vi "PIFN_System_GUI.vi"() -> ()   [LabVIEW 2019]
doc: "This example shows how to configure multiple channels and acquire waveforms from multiple channels."
uses:
  <vilib>/Utility/error.llb/DialogType.ctl
  <vilib>/Instr/_visa.llb/VISA Configure Serial Port (Instr).vi
  subVIs/SiPM_Tests_Global_Var.vi
  subVIs/Agilent_lib/Public/Configure/Trigger/Configure Trigger (Edge).vi
  subVIs/Agilent_lib/Agilent 2000 3000 X-Series.lvlib
panel:
  in  "Use Default Dir.":bool=TRUE
  out "Properties":string[](array[string])
  in  "Close Session":bool
  in  "HP8116A":refnum<visa-resource-name>="GPIB0::16::INSTR" caption="Function Generator HP8116A"
  in  "Power supply Agilent E3631A":refnum<visa-resource-name>="GPIB0::5::INSTR"
  out "Meas Ind":bool
  in  "x = y?":bool
  in  "Spectrum Only":bool
  in  "System Type":bool=TRUE
  in  "Nb_of_Events":i32 caption="Events to Record"
  in  "Abort":bool
  in  "Step Size (mm)":sgl=4.2 min=0 step=0.2
  in  "Nb of steps":u8=144
  in  "Nb of Events per step":u16=100
  in  "Time to Run (s)":dbl
  in  "System Settings":bool
  in  "Load file to display":bool
  in  "Calibration Tests":bool
  in  "Stop Button":bool
  in  "Free Run":bool
  in  "Tab Control 2":T1(tab)=enum."DPC System"
  in  "Trigger Source":T2(ring)
  in  "Input \nCoupling":T3(ring)=enum."DC Coupling"
  in  "Edge \nSlope":enum16{"Pos", "Neg", "Either", "Alt"}(ring)=enum."Neg"
  in  "Trigger Level (V)":dbl(knob)=-0.045 min=-10.0 max=10.0 step=0.01 scale=0.0..5.0
  in  "EN 4":bool
  in  "Ch 4 Vertical Scale":dbl(knob)=0.1 min=0.0 max=5.0 step=0.05 scale=0.0..5.0
  in  "CH 4  offset":dbl(knob)=-0.35 min=-10.0 max=10.0 step=0.01 scale=0.0..10.0
  in  "Ch3 Vertical Scale":dbl(knob)=0.1 min=0.0 max=5.0 step=0.05 scale=0.0..5.0
  in  "CH 3  offset":dbl(knob)=-0.35 min=-10.0 max=10.0 step=0.01 scale=0.0..10.0
  in  "EN 3":bool
  in  "EN 2":bool=TRUE
  in  "Ch 2 Vertical Scale":dbl(knob)=0.1 min=0.0 max=5.0 step=0.05 scale=0.0..5.0
  in  "CH 2  offset":dbl(knob)=-0.35 min=-10.0 max=10.0 step=0.01 scale=0.0..10.0
  in  "Ch1 Vertical Scale":dbl(knob)=0.1 min=0.0 max=5.0 step=0.001 scale=0.0..5.0
  in  "CH 1  offset":dbl(knob)=-0.35 min=-10.0 max=10.0 step=0.01 scale=0.0..10.0
  in  "EN":bool=TRUE
  in  "Agilent MSO-X 3104A \nOscilloscope":refnum<visa-resource-name>="USB0::0x0957::0x17A0::MY54100381::INSTR"
  out "Scope 2":waveform(dbl)[](graph)
  in  "Impedance":enum16{"1 MOhm", "50 Ohm"}(ring)=enum."50 Ohm"
  in  "Coupling":enum16{"AC", "DC"}(ring)=enum."DC"
  in  "Vertical Setting":enum16{"Vertical Scale", "Vertical Range"}(ring)
  in  "Vertical Range":dbl=40.0
  in  "Time per Division":dbl(knob)=1e-07 scale=0.0..1.0
  in  "Horizontal \nPosition":dbl(knob) scale=0.0..1.0
  in  "Ch1":u8=1 min=1 max=10 step=9
  in  "Ch2":u8=1 min=1 max=10 step=9
  in  "Ch3":u8=1 min=1 max=10 step=9
  in  "Ch4":u8=1 min=1 max=10 step=9
  in  "Trigger Source":T4(ring)
  out "Sync Error":bool
  in  "Nb of Laser Pulses":u8=1
  in  "Trig Delay":u8=50
  in  "Trig Width":u8=5
  in  "Delay":i16=30
  in  "Edge Det\nDisable":bool
  out "Spectrum":u16[][](graph)
  in  "Read Info":bool
  in  "Integr_dur":sgl(slide)=6.0 caption="Integration Duration (us)" min=0 max=12.75 step=0.05 scale=0.0..12.0 scale format="%#.2f"
  in  "Trigger thr (V)":sgl(slide)=0.005 min=0 max=3.3 step=0.001 scale=0.0..3.3
  out "Firmware Version":string="1"
  out "Hardware":string="1"
  out "Project":string="1"
  in  "DAQ Serial Port":refnum<visa-resource-name>="COM7"
  out "UART":bool
  in  "Download Confg":bool
  in  "SetSize":bool
  in  "FIFO pkt size":u16
  in  "RdFIFO 2":bool
  out "Buf Data":u8[](array[numeric])
  in  "FlushBuf":bool
  in  "RdFIFO":bool
  in  "Cmd ID":u8
  in  "Send CMD":bool
  in  "RdADC":bool
  out "ADC_data":u16
  in  "RdReg":bool
  in  "WrReg":bool
  out "RdReg_data":u8
  in  "WrReg_data":u8
  in  "RdReg_addr":u8
  in  "WrReg_addr":u8
  in  "RdReg 2":bool
  out "Bytes at port":u16
  out "Ch1":u16[](array[numeric])
  out "Ch4":u16[](array[numeric])
  out "Ch2":u16[](array[numeric])
  out "Ch3":u16[](array[numeric])
  in  "Tab Control":enum32{"Spectrum", "SiPM Array"}(tab)=enum."SiPM Array"
  in  "Spectrum?":bool
  in  "Bin Min (V)":dbl
  in  "Bin Max (V)":dbl=3.3
  out "XY Graph":T5(graph) caption="Spectrum"
  in  "Serial Settings":T6={"VISA resource name"="COM3", "baud rate"=9600, "data bits"=8, "parity"=enum."None", "stop bits"=10, "flow control"=0} {"flow control" items=["None"=0, "XON/XOFF"=1, "RTS/CTS"=2, "DTR/DSR"=4]; "stop bits" items=["1.0"=10, "1.5"=15, "2.0"=20]; "data bits" min=5 max=8 step=1}
  out "Y Position":dbl
  out "X position":dbl
  in  "Set Home":bool
  in  "Reset Stepper":bool
  out "Serial":string caption="Serial Monitor"
  in  "Motor Home":bool
  in  "Step (mm)":sgl min=0 step=0.2
  in  "X Back":bool
  in  "X forward":bool
  in  "Y back":bool
  in  "Y forward":bool
  out "en_channels":bool[](array[boolean])
  out "Col":dbl caption="Column Mean Fraction" format="%.2f"
  out "Row":dbl caption="Row Mean Fraction" format="%.2f"
  out "SiPM Y":i32 caption="SiPM Column"
  out "SiPM X":i32 caption="SiPM Row"
  out "Y-Home":dbl caption="Y-Home Position"
  out "X-Home":dbl caption="X-Home Position"
  out "Pulser":bool
  out "Bias":bool
  out "Power":bool
  out "Scope":bool
  out "Session Log":string
  in  "Read Temperature":bool
  out "Celcius":dbl(slide) scale=0.0..30.0
  in  "Default?":bool=TRUE
  out "Time (s)":dbl format="%.2f"
  in  "Save Results?":bool=TRUE
  in  "Set Manual Temp?":bool=TRUE
  in  "Temperature":string
  in  "Settings Button":bool
  in  "Results Directory":path=path "C:/Users/johnk/Desktop/ESA_Scintillator_Data"
  out "Events Recorded":i32
  in  "Measurement":string
  in  "File Name":string="1"
  in  "Enable\nVernier":bool
  in  "Enable \nREF \nBNC":bool
  in  "Time Base Type":i32(ring) items=["Main", "Window", "XY", "Roll"]
  # "NCSR  DEMOKRITOS\nInstitute of Nuclear and Particle Physics\nDetectors Instrumentation Laboratory"
  # "Proton-Ion-Fast Neutron Subsystem"
  # "Free Run Tests"
  # "Stepper Motor"
  # "Probe Attenuation"
  # "DAQ Configuration"
  # "Laser Position"
  # "Current Pos in SiPM Array"
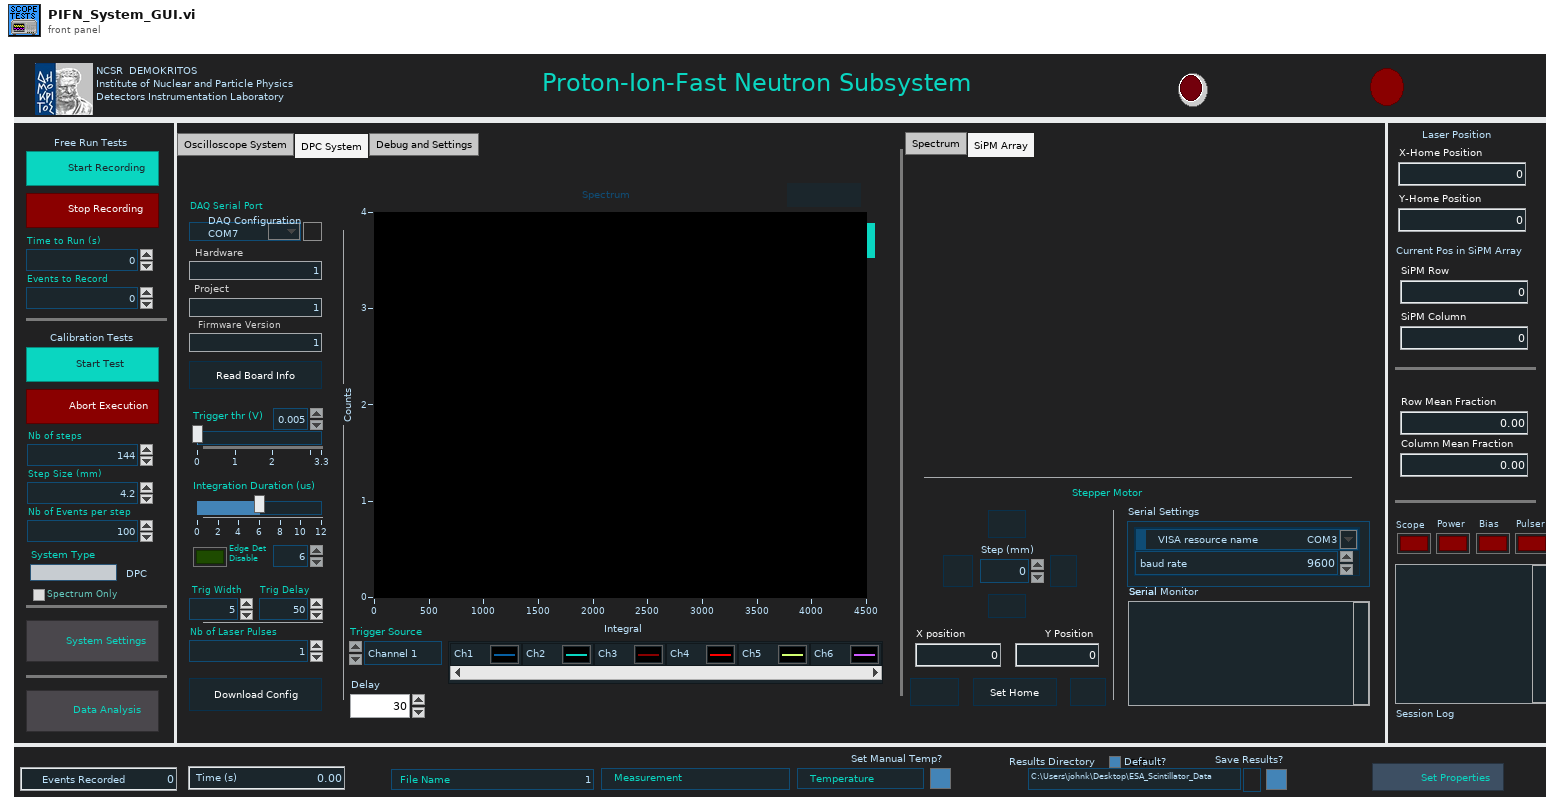
[diagram p1: front panel]
types:
  T1 = enum32{"Oscilloscope System", "DPC System", "Debug and Settings"}
  T2 = enum16{"Channel 1", "Channel 2", "Channel 3", "Channel 4", "D0", "D1", "D2", "D3", "D4", "D5", "D6", "D7", "D8", "D9", "D10", "D11", "D12", "D13", "D14", "D15", "External", "Power Line", "Waveform Generator"}
  T3 = enum16{"AC Coupling", "DC Coupling", "Low Frequency Reject"}
  T4 = enum16{"Channel 1", "Channel 2", "Channel 3", "Channel 4", "Channel 5", "Channel 6"}
  T5 = cluster{"X Values":dbl[], "Histogram: h(x)":i32[]}[]
  T6 = cluster{"VISA resource name":refnum<visa-resource-name>, "baud rate":u32, "data bits":u16, "parity":enum16{"None", "Odd", "Even", "Mark", "Space"}, "stop bits":u16, "flow control":u16}
  T7 = typedef "DialogType.ctl" = u16
  T8 = cluster{"error":bool, "code":i32, "source":string}
  T9 = enum16{"big-endian, network order", "native, host order", "little-endian"}
  T10 = enum16{"open", "open or create", "create or replace", "create", "open (read-only)"}
  T11 = cluster{"Ch1_in":dbl[], "Ch2_in":dbl[], "Ch3_in":dbl[], "Ch4_in":dbl[]}
  T12 = cluster{"Ch1":dbl[], "Ch2":dbl[], "Ch3":dbl[], "Ch4":dbl[]}
  T13 = cluster{dbl[], "mean value":dbl, dbl[], "mean value":dbl}
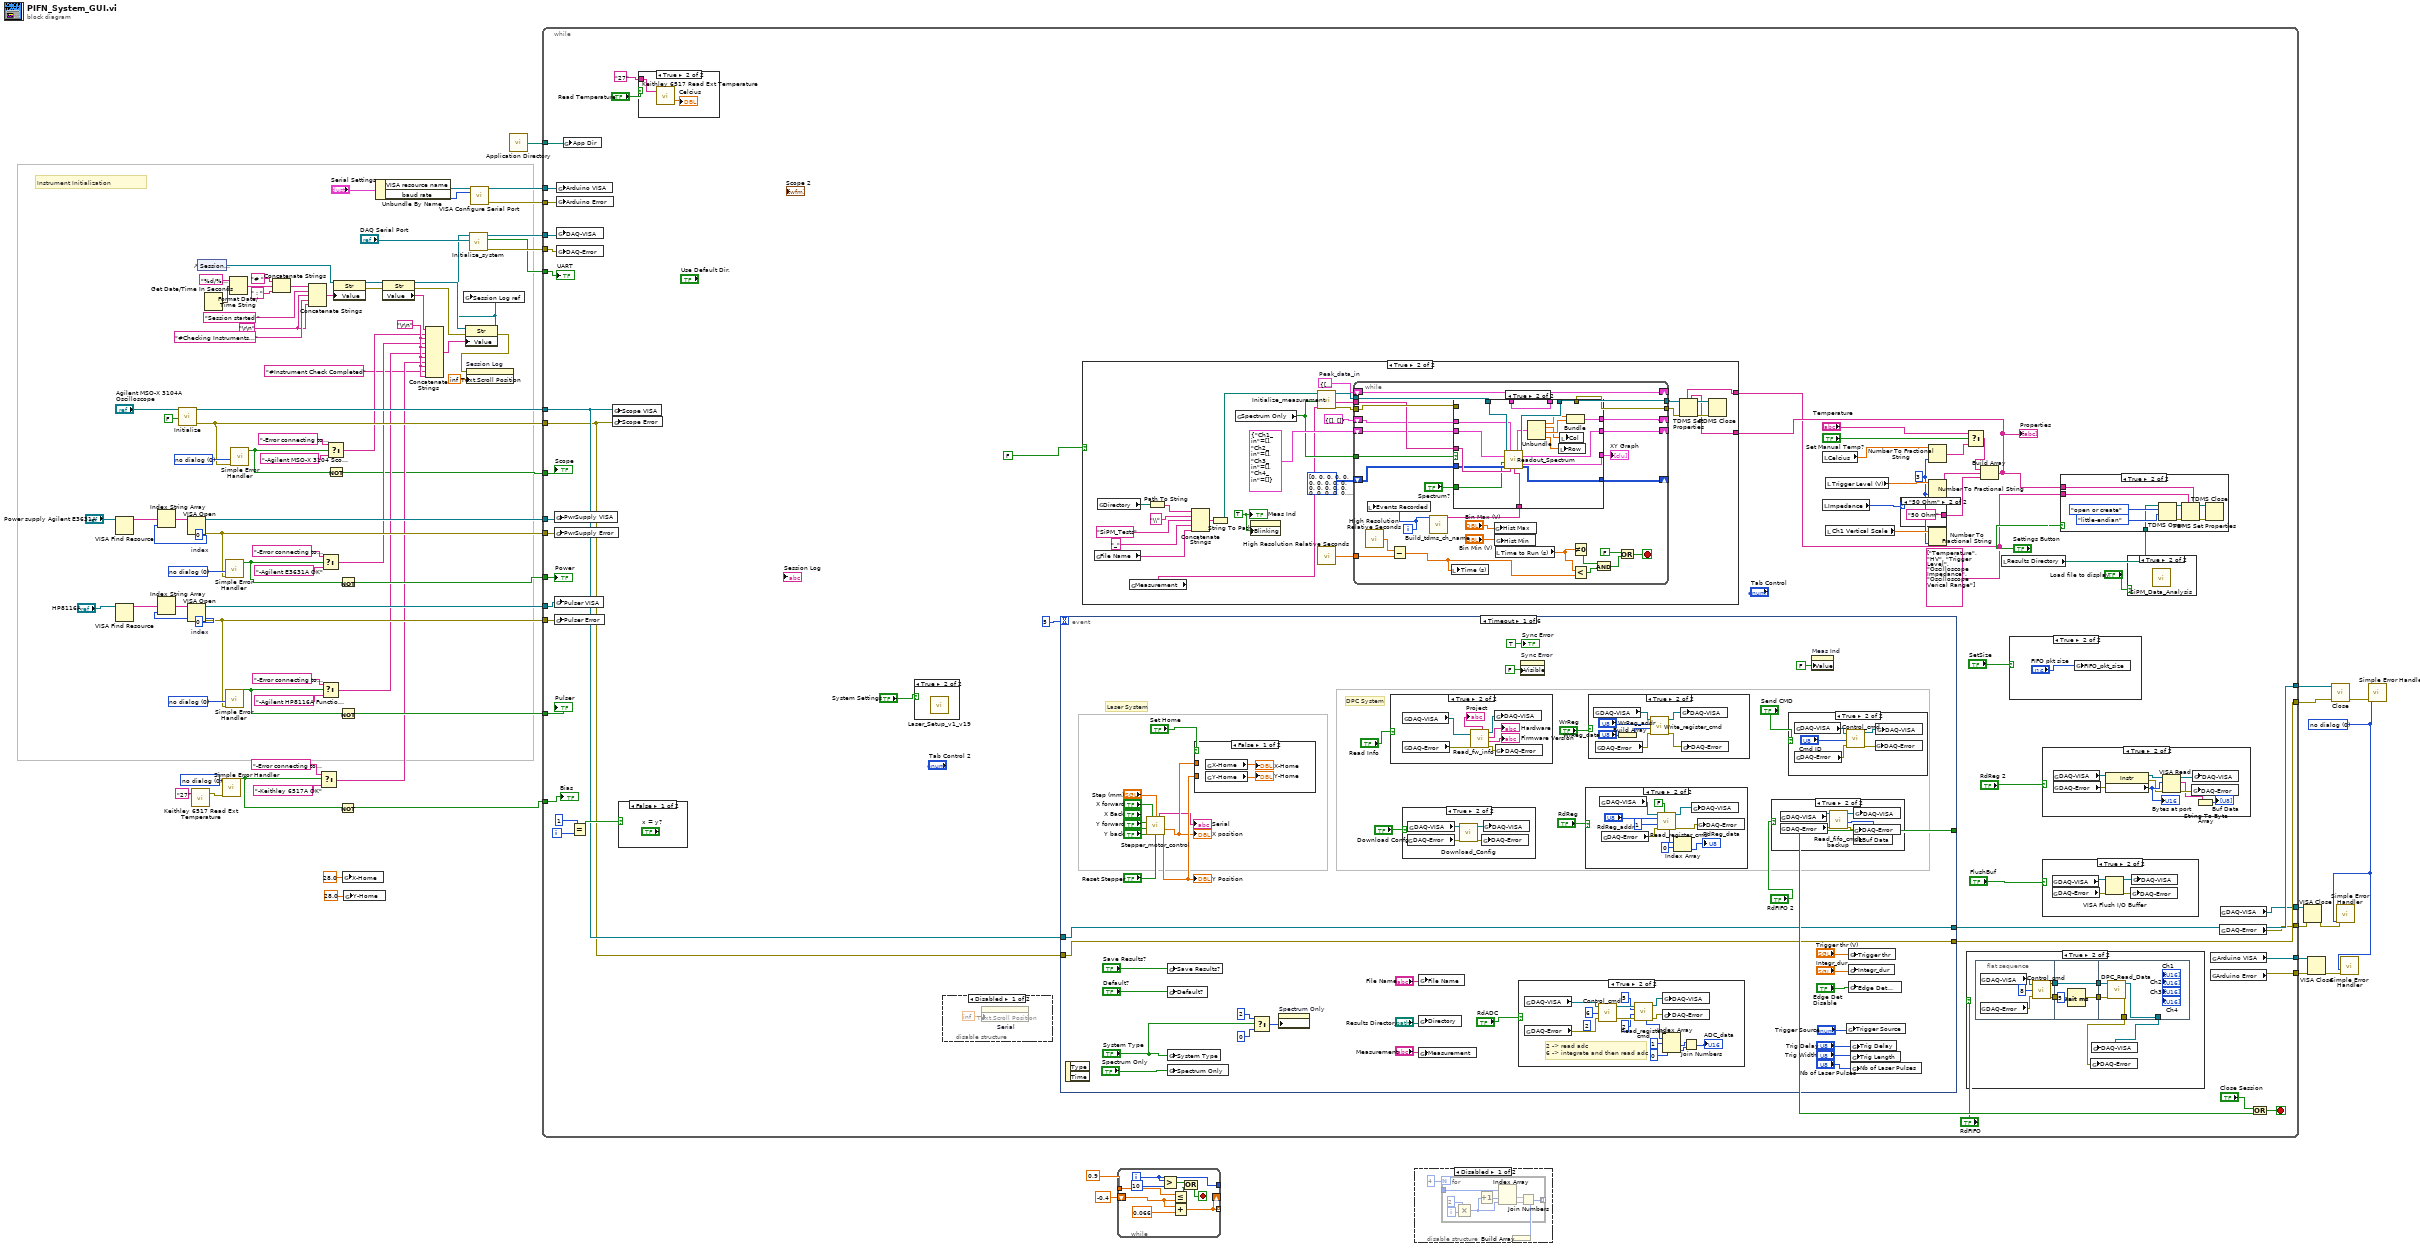
[diagram p0: block diagram]
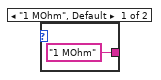
[diagram p9: hidden frame]
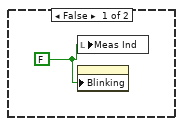
[diagram p11: hidden frame]
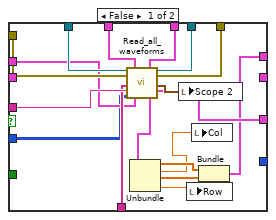
[diagram p12: hidden frame]
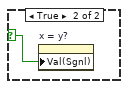
[diagram p13: hidden frame]
diagram:
  w3 = T7 0 items=["no dialog", "OK message", "continue or stop message", "OK message + warnings", "continue/stop + warnings"] ("type of dialog (OK msg:1)")
  w37 = T7 0 items=["no dialog", "OK message", "continue or stop message", "OK message + warnings", "continue/stop + warnings"] ("type of dialog (OK msg:1)")
  w48 = T7 0 items=["no dialog", "OK message", "continue or stop message", "OK message + warnings", "continue/stop + warnings"] ("type of dialog (OK msg:1)")
  w44 = 0  # index
  w53 = T7 0 items=["no dialog", "OK message", "continue or stop message", "OK message + warnings", "continue/stop + warnings"] ("type of dialog (OK msg:1)")
  w59 = 0  # index
  w65 = T7 0 items=["no dialog", "OK message", "continue or stop message", "OK message + warnings", "continue/stop + warnings"] ("type of dialog (OK msg:1)")
  w68 = "\r\n"
  w74 = "\r\n"
  w83 = FALSE ("ID Query (True)")
  # "Instrument Initialization"
  n1 = VISA Find Resource(11:"Power supply Agilent E3631A") -> (3:w58:string[])  [unwired: 2 in, 2 out]
  n2 = VISA Find Resource(11:"HP8116A") -> (3:w45:string[])  [unwired: 2 in, 2 out]
  n3 = Index String Array(1:w59, 2:w58) -> (0:w56:string)  [unwired: 1 in]
  n4 = Index String Array(1:w44, 2:w45) -> (0:w46:string)  [unwired: 1 in]
  n5 = call "Initialize.vi"("Reset (True)"=w83, "ID Query (True)"=w83, "VISA resource name"="Agilent MSO-X 3104A \nOscilloscope") -> ("error out"=w64:errorcluster, "VISA resource name out"=w87:refnum<visa-resource-name>)  [unwired: 2 in, 5 out]
  n6 = VISA Open(VISA resource name=w56) -> (VISA resource name=w55:refnum<visa-resource-name>, error out=w52:errorcluster)  [unwired: 4 in]
  n7 = VISA Open(VISA resource name=w46) -> (VISA resource name=w42:refnum<visa-resource-name>, error out=w41:errorcluster)  [unwired: 4 in]
  n8 = call "Keithley 6517 Read Ext Temperature.vi"("GPIB address"="27") -> ("error out"=w38:T8)  [unwired: 1 in, 1 out]
  n9 = control-ref of="Session Log"() -> (w70:refnum<vi>)
  n10 = Get Date/Time In Seconds() -> (seconds since 1Jan1904=w80:timestamp)
  n11 = call <vilib>:"Simple Error Handler.vi"("type of dialog (OK msg:1)"=w37, "error in (no error)"=w38) -> ("error?"=w31:bool)  [unwired: 3 in, 4 out]
  n12 = call <vilib>:"Simple Error Handler.vi"("type of dialog (OK msg:1)"=w53, "error in (no error)"=w52) -> ("error?"=w50:bool)  [unwired: 3 in, 4 out]
  n13 = call <vilib>:"Simple Error Handler.vi"("type of dialog (OK msg:1)"=w48, "error in (no error)"=w41) -> ("error?"=w29:bool)  [unwired: 3 in, 4 out]
  n14 = Format Date/Time String(time format string (%c)="%d/%m/%y_%H:%M:%S", seconds (now)=w80) -> (date/time string=w78:string)  [unwired: 1 in]
  n15 = call <vilib>:"Simple Error Handler.vi"("type of dialog (OK msg:1)"=w65, "error in (no error)"=w64) -> ("error?"=w26:bool)  [unwired: 3 in, 4 out]
  n16 = Concatenate Strings("# " ("string"), w78, " : " ("string")) -> (w77:string)
  n17 = Concatenate Strings(w77, "Session started ", w74, "#Checking Instruments..." ("string"), w74) -> (w73:string)
  n18 = Select(t="-Error connecting to Keithley 6517A" ("Session string"), s=w31, f="-Keithley 6517A OK" ("Session string")) -> (s? t:f=w33:string)
  n19 = Select(t="-Error connecting to Agilent E3631A" ("Session string"), s=w50, f="-Agilent E3631A OK" ("Session string")) -> (s? t:f=w51:string)
  n20 = Select(t="-Error connecting to HP8116A Function Generator" ("Session string"), s=w29, f="-Agilent HP8116A Function Generator OK" ("Session string")) -> (s? t:f=w40:string)
  n21 = Select(t="-Error connecting to Agilent MSO-X3104A Scope" ("Session string"), s=w26, f="-Agilent MSO-X 3104 Scope OK" ("Session string")) -> (s? t:f=w60:string)
  n22 = Not(x=w26) -> (.not. x?=w25:bool)
  n23 = property on="Property Node" class="Str"(reference=w70, "Value"=w73) -> (reference out=w72:refnum<vi>, error out=w71:errorcluster)  [unwired: 1 in]
  n24 = Not(x=w31) -> (.not. x?=w30:bool)
  n25 = Not(x=w50) -> (.not. x?=w49:bool)
  n26 = Not(x=w29) -> (.not. x?=w34:bool)
  n27 = global write "SiPM_Tests_Global_Var.vi" "X-Home"(28.0 ("X-Home")) -> ()
  n28 = global write "SiPM_Tests_Global_Var.vi" "Y-Home"(28.0 ("Y-Home")) -> ()
  n29 = Unbundle By Name("Serial Settings") -> ("VISA resource name"=w21:refnum<visa-resource-name>, "baud rate"=w22:u32)
  n30 = property on="Property Node" class="Str"(reference=w72, error in=w71) -> (reference out=w66:refnum<vi>, error out=w67:errorcluster, "Value"=w61:string)
  n31 = Concatenate Strings(w61, w60, w68, w51, w68, w40, w68, w33, w68, "#Instrument Check Completed" ("string"), w68) -> (w69:string)
  n32 = property on="Property Node" class="Str"(reference=w66, error in=w67, "Value"=w69) -> (reference out=w10:refnum<vi>, error out=w23:errorcluster)
  n33 = global write "SiPM_Tests_Global_Var.vi" "Session Log ref"(w10) -> ()
  n34 = property on="Session Log" class="Str"(error in=w23, "Text.Scroll Position"=inf) -> ()  [unwired: 1 in, 2 out]
  n35 = call "Initialize_system.vi"("Serial Port"="DAQ Serial Port", "String in"=w10) -> ("error out"=w8:errorcluster, "error?"=w7:bool, "VISA Refnum out"=w9:refnum<visa-resource-name>)  [unwired: 6 in, 1 out]
  n36 = call-poly "VISA Configure Serial Port"("VISA resource name"=w21, "baud rate (9600)"=w22) -> ("VISA resource name out"=w19:refnum<visa-resource-name>, "error out"=w18:errorcluster)  [unwired: 7 in, 5 out]
  n37 = call <vilib>:"Application Directory.vi"() -> ("Application Directory"=w14:path)
  n38 = while {
    tunnel: w87 -> [w105]
    tunnel: w64 -> [w104]
    tunnel: [w139] -> w86
    tunnel: [w138] -> w85
    tunnel: w55 -> [w109]
    tunnel: w52 -> [w108]
    tunnel: w25 -> [w113]
    tunnel: w49 -> [w112]
    tunnel: w42 -> [w107]
    tunnel: w41 -> [w106]
    tunnel: w34 -> [w111]
    tunnel: w30 -> [w110]
    tunnel: w19 -> [w102]
    tunnel: w18 -> [w103]
    tunnel: [w101] -> w16
    tunnel: [w100] -> w15
    tunnel: w14 -> [w99]
    tunnel: w9 -> [w97]
    tunnel: w8 -> [w96]
    tunnel: w7 -> [w98]
    tunnel: [w94] -> w5
    tunnel: [w93] -> w4
    i -> [w132]
    stop <- w137 stop-if-true
    w119 = string[] ["Temperature", "HV", "Trigger Level", "Oscilloscope Impedance", "Oscilloscope Verical Range"] ("property names")
    w121 = i16 3 ("precision (6)")
    n39 = global write "SiPM_Tests_Global_Var.vi" "PwrSupply VISA"(w109) -> ()
    n40 = global write "SiPM_Tests_Global_Var.vi" "PwrSupply Error"(w108) -> ()
    n41 = global write "SiPM_Tests_Global_Var.vi" "Pulser VISA"(w107) -> ()
    n42 = global write "SiPM_Tests_Global_Var.vi" "Pulser Error"(w106) -> ()
    n43 = global write "SiPM_Tests_Global_Var.vi" "Arduino VISA"(w102) -> ()
    n44 = global write "SiPM_Tests_Global_Var.vi" "Arduino Error"(w103) -> ()
    n45 = global write "SiPM_Tests_Global_Var.vi" "DAQ-VISA"(w97) -> ()
    n46 = global write "SiPM_Tests_Global_Var.vi" "DAQ-Error"(w96) -> ()
    n47 = global write "SiPM_Tests_Global_Var.vi" "App Dir"(w99) -> ()
    n48 = Equal?(x=1, y=w132) -> (x = y?=w130:bool)
    n49 = global write "SiPM_Tests_Global_Var.vi" "Scope VISA"(w105) -> ()
    n50 = global write "SiPM_Tests_Global_Var.vi" "Scope Error"(w104) -> ()
    n51 = case shown="False" w130 {
      selector: w130 -> [_ w277]
      frame False {
      }
      frame True {
        n52 = property on="x = y?" class="Bool (strict)"("Val(Sgnl)"=w277) -> ()  [unwired: 2 in, 2 out]
      }
    }
    n53 = case shown="True" "Read Temperature" {
      tunnel: "27" ("GPIB address") -> [_ w279]
      frame False {
      }
      frame True {
        n54 = call "Keithley 6517 Read Ext Temperature.vi"("GPIB address"=w279) -> ("External Temperature"=→"Celcius":dbl)  [unwired: 1 in, 1 out]
      }
    }
    n55 = case shown="True" "System Settings" {
      frame False {
      }
      frame True {
        n56 = call "Laser_Setup_v1_v19.vi"() -> ()  [unwired: 12 in]
      }
    }
    n57 = disable-structure shown="Disabled" {
      frame Disabled {
        n58 = property on="Serial" class="Str"("Text.Scroll Position"=inf) -> ()  [unwired: 2 in, 2 out]
      }
      frame Enabled {
      }
    }
    n59 = event shown="[0] Timeout" {
      selector: _ -> [_ _ _ _ _ _]
      dyn-events: _ -> [_ _ _ _ _ _]
      timeout: 5 -> [_ _ _ _ _ _]
      tunnel: w105 -> [w318 _ w425 _ _ _]
      tunnel: w104 -> [w317 _ w424 _ _ _]
      tunnel: [w318 _ w422 _ _ _] -> w139
      tunnel: [w317 _ w420 _ _ _] -> w138
      tunnel: [_ _ _ _ _ TRUE ("y")] -> w135
      event Timeout {
        # "Laser System"
        # "DPC System"
        n60 = event-data() -> ()  [unwired: 1 in, 2 out]
        n61 = call "Stepper_motor_control.vi"("X forward"="X forward", "Step Size (mm)"="Step (mm)", "X Back"="X Back", "Y forward"="Y forward", "Y back"="Y back", "Motor Home"="Reset Stepper") -> ("Serial"=→"Serial":string, "X pos"=w309:dbl, "Y pos"=w310:dbl)  [unwired: 6 in, 1 out]
        "X position" <- w309
        "Y Position" <- w310
        n62 = global write "SiPM_Tests_Global_Var.vi" "Save Results?"("Save Results?") -> ()
        n63 = global write "SiPM_Tests_Global_Var.vi" "Default?"("Default?") -> ()
        n64 = global write "SiPM_Tests_Global_Var.vi" "System Type"("System Type") -> ()
        n65 = global write "SiPM_Tests_Global_Var.vi" "Spectrum Only"("Spectrum Only") -> ()
        n66 = case shown="False" "Set Home" {
          tunnel: w309 -> [_ w375]
          tunnel: w310 -> [_ w374]
          frame False {
            n67 = global read "SiPM_Tests_Global_Var.vi" "X-Home"() -> (→"X-Home":dbl)
            n68 = global read "SiPM_Tests_Global_Var.vi" "Y-Home"() -> (→"Y-Home":dbl)
          }
          frame True {
            n69 = global write "SiPM_Tests_Global_Var.vi" "X-Home"(w375) -> ()
            n70 = global write "SiPM_Tests_Global_Var.vi" "Y-Home"(w374) -> ()
          }
        }
        n71 = Select(t=2, s="System Type", f=0) -> (s? t:f=w298:i32)
        n72 = property on="Spectrum Only" class="Bool (strict)"("DisabledEnum"=w298) -> ()  [unwired: 2 in, 2 out]
        n73 = case shown="True" "Read Info" {
          frame False {
          }
          frame True {
            n74 = global read "SiPM_Tests_Global_Var.vi" "DAQ-VISA"() -> (w366:refnum<visa-resource-name>)
            n75 = global read "SiPM_Tests_Global_Var.vi" "DAQ-Error"() -> (w365:errorcluster)
            n76 = call "Read_fw_info.vi"("error in (no error)"=w365, "VISA Refnum in"=w366) -> ("error out"=w367:errorcluster, "Firmware Version"=→"Firmware Version":string, "Hardware"=→"Hardware":string, "VISA Refnum out"=w370:refnum<visa-resource-name>, "Project"=→"Project":string)  [unwired: 5 in]
            n77 = global write "SiPM_Tests_Global_Var.vi" "DAQ-VISA"(w370) -> ()
            n78 = global write "SiPM_Tests_Global_Var.vi" "DAQ-Error"(w367) -> ()
          }
        }
        n79 = case shown="True" "Download Confg" {
          frame False {
          }
          frame True {
            n80 = global read "SiPM_Tests_Global_Var.vi" "DAQ-Error"() -> (w363:errorcluster)
            n81 = global read "SiPM_Tests_Global_Var.vi" "DAQ-VISA"() -> (w364:refnum<visa-resource-name>)
            n82 = call "Download_Config.vi"("error in"=w363, "VISA in"=w364) -> ("error out"=w361:errorcluster, "VISA Refnum out"=w362:refnum<visa-resource-name>)  [unwired: 8 in]
            n83 = global write "SiPM_Tests_Global_Var.vi" "DAQ-Error"(w361) -> ()
            n84 = global write "SiPM_Tests_Global_Var.vi" "DAQ-VISA"(w362) -> ()
          }
        }
        n85 = global write "SiPM_Tests_Global_Var.vi" "File Name"("File Name") -> ()
        n86 = global write "SiPM_Tests_Global_Var.vi" "Directory"("Results Directory") -> ()
        n87 = global write "SiPM_Tests_Global_Var.vi" "Measurement"("Measurement") -> ()
        n88 = case shown="True" "RdADC" {
          frame False {
          }
          frame True {
            (unwired) u8 2 ("Control Command")
            # "2 -> read adc\n6 -> integrate and then read adc"
            n89 = global read "SiPM_Tests_Global_Var.vi" "DAQ-VISA"() -> (w342:refnum<visa-resource-name>)
            n90 = global read "SiPM_Tests_Global_Var.vi" "DAQ-Error"() -> (w341:errorcluster)
            n91 = call "Control_cmd.vi"("Arty-7 Error In"=w341, "Control Command"=u8 6, "Arty-7 VISA In"=w342) -> ("Arty-7 Error out"=w339:errorcluster, "Arty-7 VISA out"=w340:refnum<visa-resource-name>)  [unwired: 2 in, 2 out]
            n92 = call "Read_register_cmd.vi"("Arty-7 Error In"=w339, "Words_to_read"=u16 2, "RdReg Addr"=u8 5, "Arty-7 VISA In"=w340) -> ("Arty-7 Error out"=w335:errorcluster, "Arty-7 VISA out"=w336:refnum<visa-resource-name>, "RdReg Data"=w333:u8[])  [unwired: 3 in, 2 out]
            n93 = global write "SiPM_Tests_Global_Var.vi" "DAQ-Error"(w335) -> ()
            n94 = Index Array(array=w333, index #1=1 ("index"), index #2=0 ("index")) -> (element #1=w331:u8, element #2=w330:u8)
            n95 = global write "SiPM_Tests_Global_Var.vi" "DAQ-VISA"(w336) -> ()
            n96 = Join Numbers(hi=w331, lo=w330) -> ((hi.lo)=→"ADC_data":u16)
          }
        }
        n97 = property on="Sync Error" class="Bool (strict)"("Visible"=FALSE) -> ()  [unwired: 2 in, 2 out]
        n98 = case shown="True" "RdReg" {
          frame False {
          }
          frame True {
            n99 = global read "SiPM_Tests_Global_Var.vi" "DAQ-VISA"() -> (w353:refnum<visa-resource-name>)
            n100 = global read "SiPM_Tests_Global_Var.vi" "DAQ-Error"() -> (w352:errorcluster)
            n101 = call "Read_register_cmd.vi"("Fifo-mode En"=FALSE, "Arty-7 Error In"=w352, "Words_to_read"=u16 1, "RdReg Addr"="RdReg_addr", "Arty-7 VISA In"=w353) -> ("Arty-7 Error out"=w344:errorcluster, "Arty-7 VISA out"=w345:refnum<visa-resource-name>, "RdReg Data"=w348:u8[])  [unwired: 2 in, 2 out]
            n102 = Index Array(array=w348, index=0) -> (element=→"RdReg_data":u8)
            n103 = global write "SiPM_Tests_Global_Var.vi" "DAQ-VISA"(w345) -> ()
            n104 = global write "SiPM_Tests_Global_Var.vi" "DAQ-Error"(w344) -> ()
          }
        }
        n105 = case shown="True" "WrReg" {
          frame False {
          }
          frame True {
            n106 = global read "SiPM_Tests_Global_Var.vi" "DAQ-VISA"() -> (w360:refnum<visa-resource-name>)
            n107 = global read "SiPM_Tests_Global_Var.vi" "DAQ-Error"() -> (w359:errorcluster)
            n108 = Build Array("WrReg_data") -> (w356:u8[])
            n109 = call "Write_register_cmd.vi"("Arty-7 Error In"=w359, "Data Array"=w356, "WrReg Addr"="WrReg_addr", "Arty-7 VISA In"=w360) -> ("Arty-7 Error out"=w354:errorcluster, "Arty-7 VISA out"=w355:refnum<visa-resource-name>)  [unwired: 4 in, 2 out]
            n110 = global write "SiPM_Tests_Global_Var.vi" "DAQ-VISA"(w355) -> ()
            n111 = global write "SiPM_Tests_Global_Var.vi" "DAQ-Error"(w354) -> ()
          }
        }
        n112 = case shown="True" "RdFIFO 2" {
          frame False {
          }
          frame True {
            n113 = global read "SiPM_Tests_Global_Var.vi" "DAQ-VISA"() -> (w323:refnum<visa-resource-name>)
            n114 = global read "SiPM_Tests_Global_Var.vi" "DAQ-Error"() -> (w322:errorcluster)
            n115 = call "Read_fifo_cmd_backup.vi"("error in (no error)"=w322, "VISA Refnum in"=w323) -> ("error out"=w320:errorcluster, "Data_out"=w319:u8[], "VISA Refnum out"=w321:refnum<visa-resource-name>)  [unwired: 7 in]
            n116 = global write "SiPM_Tests_Global_Var.vi" "DAQ-Error"(w320) -> ()
            n117 = local write "Buf Data"(w319) -> ()
            n118 = global write "SiPM_Tests_Global_Var.vi" "DAQ-VISA"(w321) -> ()
          }
        }
        n119 = case shown="True" "Send CMD" {
          frame False {
          }
          frame True {
            n120 = global read "SiPM_Tests_Global_Var.vi" "DAQ-VISA"() -> (w328:refnum<visa-resource-name>)
            n121 = global read "SiPM_Tests_Global_Var.vi" "DAQ-Error"() -> (w327:errorcluster)
            n122 = call "Control_cmd.vi"("Arty-7 Error In"=w327, "Control Command"="Cmd ID", "Arty-7 VISA In"=w328) -> ("Arty-7 Error out"=w326:errorcluster, "Arty-7 VISA out"=w325:refnum<visa-resource-name>)  [unwired: 2 in, 2 out]
            n123 = global write "SiPM_Tests_Global_Var.vi" "DAQ-Error"(w326) -> ()
            n124 = global write "SiPM_Tests_Global_Var.vi" "DAQ-VISA"(w325) -> ()
          }
        }
        n125 = property on="Meas Ind" class="Bool (strict)"("Value"=FALSE ("Meas Ind")) -> ()  [unwired: 2 in, 2 out]
        n126 = global write "SiPM_Tests_Global_Var.vi" "Trigger Source"("Trigger Source") -> ()
        n127 = global write "SiPM_Tests_Global_Var.vi" "Trigger thr"("Trigger thr (V)") -> ()
        n128 = global write "SiPM_Tests_Global_Var.vi" "Integr_dur"("Integr_dur") -> ()
        n129 = global write "SiPM_Tests_Global_Var.vi" "Edge Det\nDis"("Edge Det\nDisable") -> ()
        n130 = global write "SiPM_Tests_Global_Var.vi" "Trig Delay"("Trig Delay") -> ()
        n131 = global write "SiPM_Tests_Global_Var.vi" "Trig Length"("Trig Width") -> ()
        n132 = global write "SiPM_Tests_Global_Var.vi" "Nb of Laser Pulses"("Nb of Laser Pulses") -> ()
        "Sync Error" <- TRUE ("Sync Error")
      }
      event "Motor Home": Value Change {
        n133 = event-data() -> ()  [unwired: 1 in, 6 out]
        n134 = local read "Y Position"() -> (w389:dbl)
        n135 = local read "X position"() -> (w391:dbl)
        n136 = global read "SiPM_Tests_Global_Var.vi" "Y-Home"() -> (w388:dbl)
        n137 = global read "SiPM_Tests_Global_Var.vi" "X-Home"() -> (w390:dbl)
        n138 = Subtract(x=w389, y=w388) -> (x-y=w384:dbl)
        n139 = Subtract(x=w391, y=w390) -> (x-y=w387:dbl)
        n140 = Less Than 0?(x=w384) -> (x < 0?=w378:bool)
        n141 = Less Than 0?(x=w387) -> (x < 0?=w385:bool)
        n142 = Absolute Value(x=w384) -> (abs(x)=w381:dbl)
        n143 = Absolute Value(x=w387) -> (abs(x)=w386:dbl)
        n144 = flat-sequence {
          tunnel: w386 -> [w398]
          tunnel: w385 -> [w397]
          tunnel: [w395] -> w383
          tunnel: w381 -> [w394]
          tunnel: [w394] -> w379
          tunnel: w378 -> [w393]
          tunnel: [w393] -> w376
          tunnel: w383 -> [w401]
          tunnel: [w401] -> w382
          tunnel: [w400] -> w380
          tunnel: w379 -> [w400]
          tunnel: [w399] -> w377
          tunnel: w376 -> [w399]
          tunnel: w382 -> [w406]
          tunnel: w380 -> [w405]
          tunnel: w377 -> [w404]
          frame #0 {
            n145 = Not(x=w397) -> (.not. x?=w396:bool)
            n146 = call "Stepper_motor_control.vi"("X forward"=w397, "Step Size (mm)"=w398, "X Back"=w396) -> ("Serial"=w392:string, "error out"=w395:errorcluster)  [unwired: 9 in, 2 out]
            n147 = local write "Serial"(w392) -> ()
          }
          frame #1 {
            n148 = Wait (ms)(milliseconds to wait=u32 1000) -> ()  [unwired: 1 out]
          }
          frame #2 {
            n149 = Not(x=w404) -> (.not. x?=w407:bool)
            n150 = call "Stepper_motor_control.vi"("Arduino Error"=w406, "Step Size (mm)"=w405, "Y forward"=w404, "Y back"=w407) -> ("Serial"=w403:string)  [unwired: 8 in, 3 out]
            n151 = local write "Serial"(w403) -> ()
          }
        }
      }
      event "Impedance", "EN 2", "Coupling", "Vertical Range", "Vertical Setting", "Ch1 Vertical Scale", "CH 2  offset", "Ch 2 Vertical Scale", "CH 1  offset", "Enable\nVernier", "Time Base Type", "Time per Division", "Horizontal \nPosition", "Enable \nREF \nBNC", "EN", "EN 3", "CH 4  offset", "CH 3  offset", "Ch 4 Vertical Scale", "EN 4", "Ch3 Vertical Scale", "Trigger Level (V)", "Input \nCoupling", "x = y?": Value Change {
        w449 = 0 items=["Left", "Center", "Right"] ("Reference")
        w426 = 3 items=["Channel 1", "Channel 2", "Channel 3", "Channel 4"] ("Channel Name (0: Channel 1)")
        w427 = 2 items=["Channel 1", "Channel 2", "Channel 3", "Channel 4"] ("Channel Name (0: Channel 1)")
        w428 = 1 items=["Channel 1", "Channel 2", "Channel 3", "Channel 4"] ("Channel Name (0: Channel 1)")
        w429 = 0 items=["Channel 1", "Channel 2", "Channel 3", "Channel 4"] ("Channel Name (0: Channel 1)")
        n152 = event-data() -> ()  [unwired: 1 in, 1 out]
        n153 = call "Configure Channel.vi"("VISA resource name"=w425, "Vertical Scale (5.0 V)"="Ch1 Vertical Scale", "Enable Channel (T: Enable)"="EN", "Impedance (0: 1 MOhm)"="Impedance", "Channel Name (0: Channel 1)"=w429, "Coupling (1: DC)"="Coupling", "Vertical Range (40.0 V)"="Vertical Range", "error in (no error)"=w424, "Vertical Offset (0.0)"="CH 1  offset", "Probe Attenuation (1.0)"="Ch1", "Vertical Setting (1: Vertical Range)"="Vertical Setting") -> ("VISA resource name out"=w437:refnum<visa-resource-name>, "error out"=w436:errorcluster)  [unwired: 3 out]
        n154 = call "Configure Channel.vi"("VISA resource name"=w437, "Vertical Scale (5.0 V)"="Ch 2 Vertical Scale", "Enable Channel (T: Enable)"="EN 2", "Impedance (0: 1 MOhm)"="Impedance", "Channel Name (0: Channel 1)"=w428, "Coupling (1: DC)"="Coupling", "Vertical Range (40.0 V)"="Vertical Range", "error in (no error)"=w436, "Vertical Offset (0.0)"="CH 2  offset", "Probe Attenuation (1.0)"="Ch2", "Vertical Setting (1: Vertical Range)"="Vertical Setting") -> ("VISA resource name out"=w435:refnum<visa-resource-name>, "error out"=w434:errorcluster)  [unwired: 3 out]
        n155 = call "Configure Channel.vi"("VISA resource name"=w435, "Vertical Scale (5.0 V)"="Ch3 Vertical Scale", "Enable Channel (T: Enable)"="EN 3", "Impedance (0: 1 MOhm)"="Impedance", "Channel Name (0: Channel 1)"=w427, "Coupling (1: DC)"="Coupling", "Vertical Range (40.0 V)"="Vertical Range", "error in (no error)"=w434, "Vertical Offset (0.0)"="CH 3  offset", "Probe Attenuation (1.0)"="Ch3", "Vertical Setting (1: Vertical Range)"="Vertical Setting") -> ("VISA resource name out"=w433:refnum<visa-resource-name>, "error out"=w432:errorcluster)  [unwired: 3 out]
        n156 = call "Configure Channel.vi"("VISA resource name"=w433, "Vertical Scale (5.0 V)"="Ch 4 Vertical Scale", "Enable Channel (T: Enable)"="EN 4", "Impedance (0: 1 MOhm)"="Impedance", "Channel Name (0: Channel 1)"=w426, "Coupling (1: DC)"="Coupling", "Vertical Range (40.0 V)"="Vertical Range", "error in (no error)"=w432, "Vertical Offset (0.0)"="CH 4  offset", "Probe Attenuation (1.0)"="Ch4", "Vertical Setting (1: Vertical Range)"="Vertical Setting") -> ("VISA resource name out"=w431:refnum<visa-resource-name>, "error out"=w430:errorcluster)  [unwired: 3 out]
        n157 = Multiply(x="Time per Division", y=10.0) -> ()  [unwired: 1 out]
        n158 = call "Configure Timebase (Basic).vi"("VISA resource name"=w431, "Reference (1: Center)"=w449, "Enable Vernier (F: Disable)"="Enable\nVernier", "Time Base Type (0: Main)"="Time Base Type", "Scale (50 s/div)"="Time per Division", "error in (no error)"=w430, "Position (0.0)"="Horizontal \nPosition", "Enable REF BNC (F: Disable)"="Enable \nREF \nBNC") -> ("VISA resource name out"=w423:refnum<visa-resource-name>, "error out"=w421:errorcluster)  [unwired: 1 in, 5 out]
        n159 = Build Array("EN", "EN 2", "EN 3", "EN 4") -> (→"en_channels":bool[])
        n160 = call-poly "Configure Trigger.vi"("Edge Slope (0: Positive)"="Edge \nSlope", "Input Coupling (0: AC Coupling)"="Input \nCoupling", "error in (no error)"=w421, "Trigger Level (0 V)"="Trigger Level (V)", "Trigger Source (0: Channel 1)"="Trigger Source", "VISA resource name"=w423) -> ("error out"=w420:errorcluster, "VISA resource name out"=w422:refnum<visa-resource-name>)  [unwired: 4 in]
      }
      event "Calibration Tests": Value Change {
        n161 = event-data() -> ()  [unwired: 1 in, 6 out]
        n162 = flat-sequence {
          tunnel: [w484] -> w479
          tunnel: "Nb of Events per step" -> [w484]
          tunnel: [w492] -> w476
          tunnel: "Nb of steps" -> [w492]
          tunnel: [w491] -> w473
          tunnel: [w490] -> w472
          tunnel: [w489] -> w469
          tunnel: [w486] -> w465
          tunnel: [w483] -> w464
          tunnel: [w482] -> w463
          tunnel: [i32[][] [[0, 0, 0, 0, 0, 0, 0, 0, 0, 0, 0, 0], [0, 0, 0, 0, 0, 0, 0, 0, 0, 0, 0, 0], [0, 0, 0, 0, 0, 0, 0, 0, 0, 0, 0, 0], [0, 0, 0, 0, 0, 0, 0, 0, 0, 0, 0, 0], [0, 0, 0, 0, 0, 0, 0, 0, 0, 0, 0, 0], [0, 0, 0, 0, 0, 0, 0, 0, 0, 0, 0, 0], [0, 0, 0, 0, 0, 0, 0, 0, 0, 0, 0, 0], [0, 0, 0, 0, 0, 0, 0, 0, 0, 0, 0, 0], [0, 0, 0, 0, 0, 0, 0, 0, 0, 0, 0, 0], [0, 0, 0, 0, 0, 0, 0, 0, 0, 0, 0, 0], [0, 0, 0, 0, 0, 0, 0, 0, 0, 0, 0, 0], [0, 0, 0, 0, 0, 0, 0, 0, 0, 0, 0, 0]] ("Array")] -> w459
          tunnel: "Nb of Events per step" -> [w480]
          tunnel: w479 -> [w501]
          tunnel: [w501] -> w478
          tunnel: [w500] -> w477
          tunnel: w476 -> [w500]
          tunnel: [w499] -> w474
          tunnel: w473 -> [w499]
          tunnel: w472 -> [w498]
          tunnel: [w498] -> w471
          tunnel: [w497] -> w470
          tunnel: w469 -> [w497]
          tunnel: [w496] -> w466
          tunnel: w465 -> [w496]
          tunnel: w464 -> [w495]
          tunnel: w463 -> [w494]
          tunnel: [w495] -> w462
          tunnel: [w494] -> w461
          tunnel: [w493] -> w460
          tunnel: w459 -> [w493]
          tunnel: w478 -> [w513]
          tunnel: w477 -> [w506]
          tunnel: w474 -> [w511]
          tunnel: w471 -> [w510]
          tunnel: w470 -> [w509]
          tunnel: [w508] -> w468
          tunnel: [w507] -> w467
          tunnel: w466 -> [w505]
          tunnel: w462 -> [w504]
          tunnel: w461 -> [w503]
          tunnel: w460 -> [w502]
          tunnel: w468 -> [w648]
          tunnel: w467 -> [w647]
          frame #0 {
            # "Initialize Measurement"
            n163 = global write "SiPM_Tests_Global_Var.vi" "Nb of Laser Pulses"(w480) -> ()
            n164 = global read "SiPM_Tests_Global_Var.vi" "System Type"() -> (w486:bool)
            n165 = global read "SiPM_Tests_Global_Var.vi" "DAQ-Error"() -> (w482:errorcluster)
            n166 = global read "SiPM_Tests_Global_Var.vi" "DAQ-VISA"() -> (w483:refnum<visa-resource-name>)
            n167 = local write "SiPM X"(1 ("SiPM X")) -> ()
            n168 = local write "SiPM Y"(1 ("SiPM Y")) -> ()
            n169 = call "Initialize_Characterization_Tests.vi"("Evnts_per_step"=w484, "Free_run_en"=FALSE) -> ("Group_Name"=w489:string, "error out"=w490:errorcluster, "Refnum out"=w491:refnum<k34>)  [unwired: 6 in]
          }
          frame #1 {
            # "Start DAQ"
          }
          frame #2 {
            # "Run Measurements"
            n170 = for {
              N: w506 -> [_]
              tunnel: w513 -> [w545]
              tunnel: [FALSE] -> w512
              tunnel: w511 -> [w536]
              tunnel: w510 -> [w535]
              tunnel: w509 -> [w533]
              tunnel: [w528] -> w508
              tunnel: [w527] -> w507
              tunnel: w506 -> [w526]
              tunnel: w505 -> [w522]
              tunnel: w504 -> [w521]
              tunnel: w503 -> [w520]
              shift-right: [w516] -> _
              shift-left: w502 -> [w517]
              i -> [w543]
              stop <- w542 stop-if-true
              n171 = flat-sequence {
                tunnel: w545 -> [w558]
                tunnel: [w558] -> w540
                tunnel: [w555] -> w538
                tunnel: [w554] -> w537
                tunnel: w536 -> [w554]
                tunnel: w535 -> [w553]
                tunnel: [w553] -> w534
                tunnel: w533 -> [_]
                tunnel: [w552] -> w523
                tunnel: w522 -> [w552]
                tunnel: w521 -> [w551]
                tunnel: w520 -> [w547]
                tunnel: [w549] -> w519
                tunnel: [w548] -> w518
                tunnel: [w573] -> w544
                tunnel: [w572] -> w542
                tunnel: w540 -> [w574]
                tunnel: w538 -> [w571]
                tunnel: w537 -> [w570]
                tunnel: w534 -> [w569]
                tunnel: [w568] -> w532
                tunnel: [w567] -> w530
                tunnel: [w566] -> w525
                tunnel: w523 -> [w565]
                tunnel: w519 -> [w564]
                tunnel: w518 -> [w563]
                tunnel: w517 -> [w562]
                tunnel: [w561] -> w516
                tunnel: [w560] -> w515
                tunnel: [w559] -> w514
                tunnel: w544 -> [w627]
                tunnel: w543 -> [w623]
                tunnel: [w627] -> w541
                tunnel: w532 -> [w626]
                tunnel: [w626] -> w531
                tunnel: w530 -> [w625]
                tunnel: [w625] -> w529
                tunnel: w526 -> [w622]
                tunnel: w525 -> [w621]
                tunnel: [w621] -> w524
                tunnel: w515 -> [w619]
                tunnel: w514 -> [w618]
                tunnel: [w643] -> _
                tunnel: w541 -> [w643]
                tunnel: w531 -> [w641]
                tunnel: w529 -> [w640]
                tunnel: [w641] -> w528
                tunnel: [w640] -> w527
                tunnel: w524 -> [w639]
                tunnel: [w639] -> _
                frame #0 {
                  # "Start DAQ"
                  # "Settling Time"
                  n172 = local read "SiPM X"() -> (w557:i32)
                  n173 = local read "SiPM Y"() -> (w556:i32)
                  n174 = call "Control_cmd.vi"("Arty-7 Error In"=w547, "Control Command"=u8 3, "Arty-7 VISA In"=w551) -> ("Arty-7 Error out"=w548:errorcluster, "Arty-7 VISA out"=w549:refnum<visa-resource-name>)  [unwired: 2 in, 2 out]
                  n175 = Wait (ms)(milliseconds to wait=u32 800) -> ()  [unwired: 1 out]
                  n176 = call "Build_tdms_group_name.vi"("SiPM Y"=w556, "SiPM X"=w557) -> ("Group_name"=w555:string)  [unwired: 9 in]
                }
                frame #1 {
                  # "Send Laser Pulse & Acquire Measurement"
                  n177 = case shown="True" w565 {
                    tunnel: w574 -> [w584 _]
                    tunnel: [w583 _] -> w573
                    tunnel: [w582 w617] -> w572
                    tunnel: w571 -> [w581 _]
                    tunnel: w570 -> [w580 w611]
                    tunnel: w569 -> [w579 w610]
                    tunnel: [w578 w609] -> w568
                    tunnel: [w577 _] -> w567
                    tunnel: [w576 _] -> w566
                    tunnel: w564 -> [_ w615]
                    tunnel: w563 -> [_ w614]
                    tunnel: w562 -> [w575 w606]
                    tunnel: [w575 w606] -> w561
                    tunnel: [_ w608] -> w560
                    tunnel: [_ w607] -> w559
                    frame False {
                      n178 = for {
                        N: w584 -> [_]
                        shift-right: [w600] -> w583
                        shift-left: _ -> [w601]
                        tunnel: ["Abort"] -> w582
                        tunnel: w581 -> [w596]
                        tunnel: w580 -> [w595]
                        tunnel: w579 -> [w594]
                        tunnel: [w593] -> w578
                        tunnel: [w592] -> w577
                        shift-right: [w587] -> w576
                        shift-left: _ -> [w591]
                        i -> [w598]
                        stop <- "Abort" stop-if-true
                        n179 = call "Build_tdms_ch_name.vi"("Event_nb"=w598) -> ("Channel_name"=w597:string[])  [unwired: 10 in]
                        n180 = call "Read_all_waveforms.vi"("tdms file in"=w595, "error in"=w594, "Channel names"=w597, "Group name"=w596, "Peak_data_in"=w601, "In_cluster"=w591) -> ("Peak_data_out"=w600:T12, "Out_Cluster"=w590:T13, "tdms file out"=w593:refnum<k34>, "error out"=w592:errorcluster, "Waveforms"=w603:waveform(dbl)[], "Spectrum"=w602:T5)  [unwired: 7 in, 1 out]
                        n181 = Unbundle(w590) -> (w589:dbl[], "mean value"=→"Col":dbl, w588:dbl[], "mean value"=→"Row":dbl)
                        n182 = local write "Scope 2"(w603) -> ()
                        n183 = local write "XY Graph"(w602) -> ()
                        n184 = Bundle(w589, w588) -> (w587:cluster{dbl[], dbl[]})  [unwired: 1 in]
                      }
                    }
                    frame True {
                      # "2"
                      # "1"
                      n185 = call "Control_cmd.vi"("Arty-7 Error In"=w614, "Control Command"=u8 5, "Arty-7 VISA In"=w615) -> ("Arty-7 Error out"=w613:errorcluster, "Arty-7 VISA out"=w612:refnum<visa-resource-name>)  [unwired: 2 in, 2 out]
                      n186 = local read "Abort"() -> (w617:bool)
                      n187 = call "DPC_Read_Data.vi"("error in"=w613, "VISA in"=w612) -> ("error out"=w607:errorcluster, "DataOut"=w604:u16[][], "VISA out"=w608:refnum<visa-resource-name>)  [unwired: 6 in, 1 out]
                      n188 = call "DPC_Plot_Data.vi"("error in"=w610, "DataIn"=w604, "tdms file in"=w611) -> ("Sreg_Out"=w605:u16[][], "tdms file out"=w609:refnum<k34>)  [unwired: 2 in, 1 out]
                      n189 = local write "Spectrum"(w605) -> ()
                    }
                  }
                }
                frame #2 {
                  # "Stop DAQ"
                  # "Move to Next Position"
                  n190 = Not Equal?(x=w623, y=w622) -> (x != y?=w624:bool)
                  n191 = case shown="True" w624 {
                    tunnel: w623 -> [_ w633]
                    frame False {
                      # "Do nothing if this is\nthe last step"
                    }
                    frame True {
                      n192 = call "Current_SiPM_position.vi"("Iteration"=w633) -> ("SiPM_X"=→"SiPM X":i32, "Boolean 2"=w632:bool, "Boolean"=w630:bool, "SiPM_Y"=→"SiPM Y":i32)  [unwired: 7 in]
                      n193 = case shown="True" w632 {
                        tunnel: "Step Size (mm)" -> [w636 w637]
                        tunnel: w630 -> [w635 _]
                        frame False {
                          # "Move X"
                          n194 = Not(x=w635) -> (.not. x?=w634:bool)
                          n195 = call "Stepper_motor_move.vi"("X forward"=w635, "Step Size (mm)"=w636, "X Back"=w634) -> ()  [unwired: 12 in, 1 out]
                        }
                        frame True {
                          # "Move Y"
                          n196 = call "Stepper_motor_move.vi"("Step Size (mm)"=w637, "Y forward"=TRUE) -> ()  [unwired: 13 in, 1 out]
                        }
                      }
                    }
                  }
                  n197 = call "Control_cmd.vi"("Arty-7 Error In"=w618, "Control Command"=u8 4, "Arty-7 VISA In"=w619) -> ()  [unwired: 2 in, 4 out]
                }
                frame #3 {
                  # "Delay Time"
                  n198 = Wait (ms)(milliseconds to wait=u32 2500) -> ()  [unwired: 1 out]
                }
              }
            }
            n199 = local write "Abort"(w512) -> ()
          }
          frame #3 {
            # "Close Measurement"
            n200 = local read "Properties"() -> (w644:string[])
            n201 = TDMS Set Properties(5:w644, 7:string[] ["Temperature", "HV", "Trigger Level", "Oscilloscope Impedance", "Oscilloscope Verical Range"] ("property names"), 8:w647, 11:w648) -> (0:w646:errorcluster, 3:w649:refnum<k34>)  [unwired: 2 in, 2 out]
            n202 = call "Done"() -> ()  [unwired: 10 in, 2 out]
            n203 = TDMS Close(8:w646, 11:w649) -> ()  [unwired: 2 out]
          }
        }
      }
      event "Free Run": Value Change {
        w651 = T7 0 items=["no dialog", "OK message", "continue or stop message", "OK message + warnings", "continue/stop + warnings"] ("type of dialog (OK msg:1)")
        n204 = event-data() -> ()  [unwired: 1 in, 1 out]
        n205 = global read "SiPM_Tests_Global_Var.vi" "System Type"() -> (w665:bool)
        n206 = global read "SiPM_Tests_Global_Var.vi" "DAQ-Error"() -> (w667:errorcluster)
        n207 = global read "SiPM_Tests_Global_Var.vi" "DAQ-VISA"() -> (w668:refnum<visa-resource-name>)
        n208 = flat-sequence {
          tunnel: w668 -> [w684]
          tunnel: w667 -> [w683]
          tunnel: [w682] -> w666
          tunnel: w665 -> [w682]
          tunnel: [w678] -> w664
          tunnel: [w677] -> w663
          tunnel: [w676] -> w660
          tunnel: w666 -> [w696]
          tunnel: w664 -> [w694]
          tunnel: w663 -> [w693]
          tunnel: [w692] -> w662
          tunnel: [w691] -> w661
          tunnel: w660 -> [w686]
          tunnel: w662 -> [w747]
          tunnel: w661 -> [w746]
          tunnel: [w745] -> w658
          tunnel: [w744] -> w657
          frame #0 {
            # "Initialize Measurement"
            # "Download\nConfig"
            # "Start \nDAQ"
            n209 = global read "SiPM_Tests_Global_Var.vi" "Nb of Laser Pulses"() -> (w676:u8)
            n210 = call "Download_Config.vi"("error in"=w683, "VISA in"=w684) -> ("error out"=w681:errorcluster, "VISA Refnum out"=w680:refnum<visa-resource-name>)  [unwired: 8 in]
            n211 = call "Control_cmd.vi"("Arty-7 Error In"=w681, "Control Command"=u8 3, "Arty-7 VISA In"=w680) -> ("Arty-7 Error out"=w677:errorcluster, "Arty-7 VISA out"=w678:refnum<visa-resource-name>)  [unwired: 2 in, 2 out]
          }
          frame #1 {
            # "Run Measurements"
            n212 = call "Initialize_Characterization_Tests.vi"("Evnts_per_step"=w686, "Free_run_en"=TRUE) -> ("Group_Name"=w689:string, "error out"=w688:errorcluster, "Refnum out"=w687:refnum<k34>)  [unwired: 6 in]
            n213 = call <vilib>:"High Resolution Relative Seconds.vi"() -> ("relative seconds"=w695:dbl)
            n214 = case shown="True" w696 {
              tunnel: w695 -> [_ w705]
              tunnel: w694 -> [_ w704]
              tunnel: w693 -> [_ w703]
              tunnel: w687 -> [_ w702]
              tunnel: w688 -> [_ w701]
              tunnel: w689 -> [_ w700]
              tunnel: [_ w699] -> w692
              tunnel: [_ w698] -> w691
              tunnel: u16[][] array6x4096[24576 elements] ("DataIn") -> [_ w697]
              frame False {
              }
              frame True {
                n215 = while {
                  tunnel: w705 -> [w731]
                  tunnel: w704 -> [w716]
                  tunnel: w703 -> [w715]
                  tunnel: w702 -> [_]
                  tunnel: w701 -> [_]
                  tunnel: w700 -> [_]
                  tunnel: [w711] -> w699
                  tunnel: [w710] -> w698
                  shift-right: [w707] -> _
                  shift-left: w697 -> [w708]
                  i -> [w717]
                  stop <- w721 stop-if-true
                  # "Send Laser Pulse"
                  # "Process Data"
                  # "Read Data"
                  n216 = disable-structure shown="Enabled" {
                    disable-tunnel: w716 -> [w741 w743]
                    disable-tunnel: w715 -> [w740 w742]
                    disable-tunnel: [w738 w743] -> w713
                    disable-tunnel: [w737 w742] -> w712
                    frame Enabled {
                      n217 = call "Control_cmd.vi"("Arty-7 Error In"=w740, "Control Command"=u8 5, "Arty-7 VISA In"=w741) -> ("Arty-7 Error out"=w737:errorcluster, "Arty-7 VISA out"=w738:refnum<visa-resource-name>)  [unwired: 2 in, 2 out]
                    }
                    frame Disabled {
                    }
                  }
                  n218 = call <vilib>:"High Resolution Relative Seconds.vi"() -> ("relative seconds"=w732:dbl)
                  n219 = Number To Decimal String(number=w717) -> (decimal integer string=w719:string)  [unwired: 1 in]
                  n220 = Subtract(x=w732, y=w731) -> (x-y=w728:dbl)
                  "Time (s)" <- w728
                  n221 = call "DPC_Read_Data.vi"("error in"=w712, "VISA in"=w713) -> ("error out"=w710:errorcluster, "DataOut"=w709:u16[][], "VISA out"=w711:refnum<visa-resource-name>, "Error"=w706:bool)  [unwired: 6 in]
                  n222 = Not Equal To 0?(x="Nb_of_Events") -> (x != 0?=w725:bool)
                  n223 = Less?(x="Nb_of_Events", y=w717) -> (x < y?=w724:bool)
                  n224 = Not Equal To 0?(x="Time to Run (s)") -> (x != 0?=w729:bool)
                  n225 = Less?(x="Time to Run (s)", y=w728) -> (x < y?=w730:bool)
                  n226 = Concatenate Strings("Event#", w719) -> ()  [unwired: 1 out]
                  n227 = property on="Sync Error" class="Bool (strict)"("Visible"=w706) -> ()  [unwired: 2 in, 2 out]
                  n228 = And(x=w725, y=w724) -> (x .and. y?=w722:bool)
                  n229 = And(x=w729, y=w730) -> (x .and. y?=w726:bool)
                  n230 = Compound Arithmetic op=OR(w722, w726, "Stop Button") -> (w721:bool)
                  n231 = case shown="True" w706 {
                    tunnel: w709 -> [w735 _]
                    tunnel: w708 -> [w734 w736]
                    tunnel: [w733 w736] -> w707
                    frame False {
                      n232 = call "DPC_Plot_Data.vi"("Sreg_In"=w734, "DataIn"=w735) -> ("Sreg_Out"=w733:u16[][])  [unwired: 3 in, 2 out]
                    }
                    frame True {
                    }
                  }
                  "Spectrum" <- w707
                  n233 = Wait (ms)(milliseconds to wait="Delay") -> ()  [unwired: 1 out]
                  "Events Recorded" <- w717
                }
              }
            }
          }
          frame #2 {
            # "Stop \nDAQ"
            # "Close Measurement"
            n234 = call "Control_cmd.vi"("Arty-7 Error In"=w746, "Control Command"=u8 4, "Arty-7 VISA In"=w747) -> ("Arty-7 Error out"=w744:errorcluster, "Arty-7 VISA out"=w745:refnum<visa-resource-name>)  [unwired: 2 in, 2 out]
          }
        }
        n235 = VISA Flush I/O Buffer(VISA resource name=w658, error in (no error)=w657) -> (VISA resource name out=w656:refnum<visa-resource-name>, error out=w655:errorcluster)  [unwired: 1 in]
        n236 = for {
          N: 10 -> [_]
          tunnel: w656 -> [w674]
          tunnel: w655 -> [w673]
          tunnel: [w670] -> w654
          tunnel: [w669] -> w653
          n237 = property class="Instr"(reference=w674, error in=w673) -> (reference out=w675:refnum<visa-resource-name>, error out=w671:errorcluster, "Serial Settings:Number of Bytes at Serial Port"=w672:u32)
          n238 = VISA Read(VISA resource name=w675, byte count=w672, error in (no error)=w671) -> (VISA resource name out=w670:refnum<visa-resource-name>, error out=w669:errorcluster)  [unwired: 2 out]
        }
        n239 = property on="Meas Ind" class="Bool (strict)"("Value"=TRUE ("Meas Ind")) -> ()  [unwired: 2 in, 2 out]
        n240 = call <vilib>:"Simple Error Handler.vi"("type of dialog (OK msg:1)"=w651, "error in (no error)"=w653) -> ("error out"=w652:errorcluster)  [unwired: 3 in, 4 out]
        n241 = global write "SiPM_Tests_Global_Var.vi" "DAQ-Error"(w652) -> ()
        n242 = global write "SiPM_Tests_Global_Var.vi" "DAQ-VISA"(w654) -> ()
      }
      event Panel Close {
        n243 = event-data() -> ()  [unwired: 1 in, 4 out]
      }
    }
    n244 = local read "Celcius"() -> (w125:dbl)
    n245 = local read "Impedance"() -> (w124:enum16{"1 MOhm", "50 Ohm"})
    n246 = local read "Trigger Level (V)"() -> (w129:dbl)
    n247 = local read "Ch1 Vertical Scale"() -> (w122:dbl)
    n248 = case shown="\"50 Ohm\"" w124 {
      tunnel: ["1 MOhm" "50 Ohm"] -> w123
      frame "1 MOhm", Default {
      }
      frame "50 Ohm" {
      }
    }
    n249 = Number To Fractional String(number=w125, precision (6)=w121) -> (F-format string=w118:string)  [unwired: 2 in]
    n250 = Number To Fractional String(number=w129, precision (6)=w121) -> (F-format string=w128:string)  [unwired: 2 in]
    n251 = Number To Fractional String(number=w122, precision (6)=w121) -> ()  [unwired: 2 in, 1 out]
    n252 = case shown="True" "RdFIFO" {
      frame False {
      }
      frame True {
        n253 = flat-sequence {
          tunnel: [w164] -> w162
          tunnel: [w163] -> w161
          tunnel: w162 -> [w170]
          tunnel: w161 -> [w169]
          tunnel: [w170] -> w160
          tunnel: [w169] -> w159
          tunnel: w160 -> [w173]
          tunnel: w159 -> [w174]
          tunnel: [w172] -> w158
          tunnel: [w171] -> w157
          frame #0 {
            n254 = global read "SiPM_Tests_Global_Var.vi" "DAQ-VISA"() -> (w167:refnum<visa-resource-name>)
            n255 = global read "SiPM_Tests_Global_Var.vi" "DAQ-Error"() -> (w166:errorcluster)
            n256 = call "Control_cmd.vi"("Arty-7 Error In"=w166, "Control Command"=u8 8, "Arty-7 VISA In"=w167) -> ("Arty-7 Error out"=w164:errorcluster, "Arty-7 VISA out"=w163:refnum<visa-resource-name>)  [unwired: 2 in, 2 out]
          }
          frame #1 {
            n257 = Wait (ms)(milliseconds to wait=u32 5) -> ()  [unwired: 1 out]
          }
          frame #2 {
            n258 = call "DPC_Read_Data.vi"("error in"=w173, "VISA in"=w174) -> ("error out"=w171:errorcluster, "VISA out"=w172:refnum<visa-resource-name>)  [unwired: 6 in, 2 out]
          }
        }
        n259 = global write "SiPM_Tests_Global_Var.vi" "DAQ-Error"(w157) -> ()
        n260 = global write "SiPM_Tests_Global_Var.vi" "DAQ-VISA"(w158) -> ()
      }
    }
    n261 = Select(t="Temperature", s="Set Manual Temp?", f=w118) -> (s? t:f=w116:string)
    n262 = Build Array(w116, w128, w123) -> (w120:string[])
    "Properties" <- w120
    n263 = case shown="True" FALSE {
      tunnel: w120 -> [_ w209]
      tunnel: w119 -> [_ w208]
      frame False {
        w186 = FALSE ("Meas Ind")
        n264 = local write "Meas Ind"(w186) -> ()
        n265 = property on="Meas Ind" class="Bool (strict)"("Blinking"=w186) -> ()  [unwired: 2 in, 2 out]
      }
      frame True {
        w200 = T12 {"Ch1"=[], "Ch2"=[], "Ch3"=[], "Ch4"=[]}  # Peak_data_in
        w207 = TRUE ("Measurements  ON")
        n266 = global read "SiPM_Tests_Global_Var.vi" "File Name"() -> (w194:string)
        n267 = global read "SiPM_Tests_Global_Var.vi" "Directory"() -> (w195:path)
        n268 = global read "SiPM_Tests_Global_Var.vi" "Measurement"() -> (w188:string)
        n269 = Path To String(path=w195) -> (string=w192:string)
        n270 = Concatenate Strings(w192, "\\" ("string"), "SiPM_Tests", "_", w194) -> (w193:string)
        n271 = String To Path(string=w193) -> (path=w187:path)
        n272 = global read "SiPM_Tests_Global_Var.vi" "Spectrum Only"() -> (w196:bool)
        n273 = property on="Meas Ind" class="Bool (strict)"("Blinking"=w207) -> ()  [unwired: 2 in, 2 out]
        n274 = call "Initialize_measurement.vi"("Measurement"=w188, "Spectrum Only?"=w196, "file path"=w187) -> ("error out"=w203:errorcluster, "Group Name"=w202:string, "tdms file out"=w204:refnum<k34>)  [unwired: 6 in]
        n275 = call <vilib>:"High Resolution Relative Seconds.vi"() -> ("relative seconds"=w201:dbl)
        n276 = while {
          tunnel: w204 -> [w240]
          tunnel: w203 -> [w239]
          tunnel: w196 -> [w236]
          tunnel: [w238] -> w206
          tunnel: [w237] -> w205
          tunnel: w202 -> [w235]
          tunnel: w201 -> [w230]
          shift-right: [w224] -> _
          shift-left: w200 -> [w225]
          shift-right: [w221] -> _
          shift-left: cluster{dbl[], dbl[]} {[], []} -> [w222]
          shift-right: [w219] -> _
          shift-left: T11 {"Ch1_in"=[], "Ch2_in"=[], "Ch3_in"=[], "Ch4_in"=[]} ("Ch_in") -> [w220]
          shift-right: [w212] -> _
          shift-left: i32[][] [[0, 0, 0, 0, 0, 0, 0, 0, 0, 0, 0, 0], [0, 0, 0, 0, 0, 0, 0, 0, 0, 0, 0, 0], [0, 0, 0, 0, 0, 0, 0, 0, 0, 0, 0, 0], [0, 0, 0, 0, 0, 0, 0, 0, 0, 0, 0, 0], [0, 0, 0, 0, 0, 0, 0, 0, 0, 0, 0, 0], [0, 0, 0, 0, 0, 0, 0, 0, 0, 0, 0, 0], [0, 0, 0, 0, 0, 0, 0, 0, 0, 0, 0, 0], [0, 0, 0, 0, 0, 0, 0, 0, 0, 0, 0, 0], [0, 0, 0, 0, 0, 0, 0, 0, 0, 0, 0, 0], [0, 0, 0, 0, 0, 0, 0, 0, 0, 0, 0, 0], [0, 0, 0, 0, 0, 0, 0, 0, 0, 0, 0, 0], [0, 0, 0, 0, 0, 0, 0, 0, 0, 0, 0, 0], [0, 0, 0, 0, 0, 0, 0, 0, 0, 0, 0, 0], [0, 0, 0, 0, 0, 0, 0, 0, 0, 0, 0, 0], [0, 0, 0, 0, 0, 0, 0, 0, 0, 0, 0, 0], [0, 0, 0, 0, 0, 0, 0, 0, 0, 0, 0, 0], [0, 0, 0, 0, 0, 0, 0, 0, 0, 0, 0, 0], [0, 0, 0, 0, 0, 0, 0, 0, 0, 0, 0, 0], [0, 0, 0, 0, 0, 0, 0, 0, 0, 0, 0, 0], [0, 0, 0, 0, 0, 0, 0, 0, 0, 0, 0, 0], [0, 0, 0, 0, 0, 0, 0, 0, 0, 0, 0, 0], [0, 0, 0, 0, 0, 0, 0, 0, 0, 0, 0, 0], [0, 0, 0, 0, 0, 0, 0, 0, 0, 0, 0, 0], [0, 0, 0, 0, 0, 0, 0, 0, 0, 0, 0, 0]] ("Array") -> [w218]
          i -> [w214]
          stop <- w229 stop-if-true
          n277 = call <vilib>:"High Resolution Relative Seconds.vi"() -> ("relative seconds"=w231:dbl)
          n278 = local write "Events Recorded"(w214) -> ()
          n279 = Subtract(x=w231, y=w230) -> (x-y=w216:dbl)
          n280 = call "Build_tdms_ch_name.vi"("Event_nb"=w214) -> ("Channel_name"=w223:string[])  [unwired: 10 in]
          n281 = local write "Time (s)"(w216) -> ()
          n282 = case shown="True" w236 {
            tunnel: w240 -> [w258 w276]
            tunnel: w239 -> [w257 _]
            tunnel: [w256 w275] -> w238
            tunnel: [w255 _] -> w237
            tunnel: w235 -> [w253 w274]
            tunnel: w223 -> [w252 w273]
            tunnel: [w251 w262] -> w232
            tunnel: w225 -> [w250 w272]
            tunnel: [w249 w272] -> w224
            tunnel: w222 -> [w248 w267]
            tunnel: [w246 w265] -> w221
            tunnel: w220 -> [_ w264]
            tunnel: [_ w263] -> w219
            tunnel: w218 -> [w241 w261]
            tunnel: "Spectrum?" -> [_ w260]
            tunnel: [_ w259] -> w212
            frame False {
              n283 = call "Read_all_waveforms.vi"("tdms file in"=w258, "error in"=w257, "Channel names"=w252, "Group name"=w253, "Intensity_in"=w241, "Peak_data_in"=w250, "In_cluster"=w248) -> ("Peak_data_out"=w249:T12, "Out_Cluster"=w247:T13, "tdms file out"=w256:refnum<k34>, "error out"=w255:errorcluster, "Waveforms"=w254:waveform(dbl)[], "Spectrum"=w251:T5)  [unwired: 6 in, 1 out]
              n284 = Unbundle(w247) -> (w245:dbl[], "mean value"=w243:dbl, w244:dbl[], "mean value"=w242:dbl)
              n285 = local write "Scope 2"(w254) -> ()
              n286 = local write "Row"(w242) -> ()
              n287 = local write "Col"(w243) -> ()
              n288 = Bundle(w245, w244) -> (w246:cluster{dbl[], dbl[]})  [unwired: 1 in]
            }
            frame True {
              n289 = call "Readout_Spectrum.vi"("tdms file in"=w276, "Fraction In"=w267, "Ch_in"=w264, "Spectrum?"=w260, "Intensity_in"=w261, "group name"=w274, "channel names"=w273) -> ("Fraction_out"=w266:T13, "tdms file out"=w275:refnum<k34>, "Ch_out"=w263:cluster{dbl[], dbl[], dbl[], dbl[]}, "Spectrum_out"=w262:T5, "Intensity_out"=w259:i32[][])  [unwired: 4 in]
              n290 = Unbundle(w266) -> (w271:dbl[], "mean value"=w269:dbl, w270:dbl[], "mean value"=w268:dbl)
              n291 = local write "Row"(w268) -> ()
              n292 = local write "Col"(w269) -> ()
              n293 = Bundle(w271, w270) -> (w265:cluster{dbl[], dbl[]})  [unwired: 1 in]
            }
          }
          "XY Graph" <- w232
          n294 = global write "SiPM_Tests_Global_Var.vi" "Hist Max"("Bin Max (V)") -> ()
          n295 = global write "SiPM_Tests_Global_Var.vi" "Hist Min"("Bin Min (V)") -> ()
          n296 = local read "Time to Run (s)"() -> (w215:dbl)
          n297 = Not Equal To 0?(x=w215) -> (x != 0?=w227:bool)
          n298 = Less?(x=w215, y=w216) -> (x < y?=w228:bool)
          n299 = And(x=w227, y=w228) -> (x .and. y?=w226:bool)
          n300 = Or(x=FALSE, y=w226) -> (x .or. y?=w229:bool)
        }
        n301 = TDMS Set Properties(5:w209, 7:w208, 8:w205, 11:w206) -> (0:w210:errorcluster, 3:w211:refnum<k34>)  [unwired: 2 in, 2 out]
        n302 = TDMS Close(8:w210, 11:w211) -> ()  [unwired: 2 out]
        "Meas Ind" <- w207
      }
    }
    n303 = local read "Results Directory"() -> (w126:path)
    n304 = case shown="True" "SetSize" {
      frame False {
      }
      frame True {
        n305 = global write "SiPM_Tests_Global_Var.vi" "FIFO_pkt_size"("FIFO pkt size") -> ()
      }
    }
    n306 = case shown="True" "RdReg 2" {
      frame False {
      }
      frame True {
        n307 = global read "SiPM_Tests_Global_Var.vi" "DAQ-VISA"() -> (w152:refnum<visa-resource-name>)
        n308 = global read "SiPM_Tests_Global_Var.vi" "DAQ-Error"() -> (w151:errorcluster)
        n309 = property class="Instr"(reference=w152, error in=w151) -> (reference out=w150:refnum<visa-resource-name>, error out=w148:errorcluster, "Serial Settings:Number of Bytes at Serial Port"=w149:u32)
        "Bytes at port" <- w149
        n310 = VISA Read(VISA resource name=w150, byte count=w149, error in (no error)=w148) -> (VISA resource name out=w147:refnum<visa-resource-name>, read buffer=w145:string, error out=w146:errorcluster)  [unwired: 1 out]
        n311 = global write "SiPM_Tests_Global_Var.vi" "DAQ-Error"(w146) -> ()
        n312 = global write "SiPM_Tests_Global_Var.vi" "DAQ-VISA"(w147) -> ()
        n313 = String To Byte Array(string=w145) -> (unsigned byte array=→"Buf Data":u8[])
      }
    }
    n314 = case shown="True" "FlushBuf" {
      frame False {
      }
      frame True {
        n315 = global read "SiPM_Tests_Global_Var.vi" "DAQ-VISA"() -> (w156:refnum<visa-resource-name>)
        n316 = global read "SiPM_Tests_Global_Var.vi" "DAQ-Error"() -> (w155:errorcluster)
        n317 = VISA Flush I/O Buffer(VISA resource name=w156, error in (no error)=w155) -> (VISA resource name out=w154:refnum<visa-resource-name>, error out=w153:errorcluster)  [unwired: 1 in]
        n318 = global write "SiPM_Tests_Global_Var.vi" "DAQ-Error"(w153) -> ()
        n319 = global write "SiPM_Tests_Global_Var.vi" "DAQ-VISA"(w154) -> ()
      }
    }
    n320 = case shown="True" "Settings Button" {
      tunnel: w120 -> [_ w179]
      tunnel: w119 -> [_ w178]
      tunnel: w126 -> [_ w177]
      frame False {
      }
      frame True {
        n321 = TDMS Open(9:T9."little-endian" ("byte order (2:little-endian)"), 10:T10."open or create" ("operation (0:open)"), 11:w177) -> (0:w180:errorcluster, 3:w183:refnum<k34>)  [unwired: 4 in]
        n322 = TDMS Set Properties(5:w179, 7:w178, 8:w180, 11:w183) -> (0:w181:errorcluster, 3:w182:refnum<k34>)  [unwired: 2 in, 2 out]
        n323 = TDMS Close(8:w181, 11:w182) -> ()  [unwired: 2 out]
      }
    }
    n324 = case shown="True" "Load file to display" {
      frame False {
      }
      frame True {
        n325 = call "SiPM_Data_Analysis.vi"() -> ()  [unwired: 12 in]
      }
    }
    n326 = global read "SiPM_Tests_Global_Var.vi" "Arduino Error"() -> (w100:errorcluster)
    n327 = global read "SiPM_Tests_Global_Var.vi" "Arduino VISA"() -> (w101:refnum<visa-resource-name>)
    n328 = global read "SiPM_Tests_Global_Var.vi" "DAQ-Error"() -> (w93:errorcluster)
    n329 = global read "SiPM_Tests_Global_Var.vi" "DAQ-VISA"() -> (w94:refnum<visa-resource-name>)
    n330 = Or(x="Close Session", y=w135) -> (x .or. y?=w137:bool)
    "Scope" <- w113
    "Power" <- w112
    "Bias" <- w110
    "Pulser" <- w111
    "UART" <- w98
  }
  n331 = while {
    tunnel: 0.9 ("Numeric") -> [w758]
    shift-right: [w750] -> _
    shift-left: -0.4 -> [w757]
    tunnel: [w753] -> _
    tunnel: [w750] -> _ mode=indexing
    i -> [w753]
    stop <- w751 stop-if-true
    n332 = Greater?(x=w753, y=10) -> (0:w754:bool)
    n333 = Less Or Equal?(x=w758, y=w757) -> (x <= y?=w755:bool)
    n334 = Add(x=w757, y=0.066) -> (x+y=w750:dbl)
    n335 = Or(x=w754, y=w755) -> (x .or. y?=w751:bool)
  }
  n336 = disable-structure shown="Disabled" {
    frame Disabled {
      n337 = for {
        N: 4 -> [_]
        tunnel: _ -> [w768]
        tunnel: [w761] -> w759 mode=indexing
        i -> [w767]
        n338 = Multiply(x=2, y=w767) -> (x*y=w765:i32)
        n339 = Increment(x=w765) -> (x+1=w764:i32)
        n340 = Index Array(array=w768, index #1=w764, index #2=w765) -> (element #1=w762, element #2=w763)
        n341 = Join Numbers(hi=w762, lo=w763) -> ((hi.lo)=w761:u32)
      }
      n342 = Build Array(w759) -> ()  [unwired: 1 out]
    }
    frame Enabled {
    }
  }
  n343 = VISA Close(VISA resource name=w5, error in (no error)=w4) -> (error out=w6:errorcluster)
  n344 = VISA Close(VISA resource name=w16, error in (no error)=w15) -> (error out=w17:errorcluster)
  n345 = call "Close.vi"("error in (no error)"=w85, "VISA resource name"=w86) -> ("error out"=w88:errorcluster)  [unwired: 9 out]
  n346 = call <vilib>:"Simple Error Handler.vi"("type of dialog (OK msg:1)"=w3, "error in (no error)"=w6) -> ()  [unwired: 8 out]
  n347 = call <vilib>:"Simple Error Handler.vi"("type of dialog (OK msg:1)"=w3, "error in (no error)"=w17) -> ()  [unwired: 8 out]
  n348 = call <vilib>:"Simple Error Handler.vi"("type of dialog (OK msg:1)"=w3, "error in (no error)"=w88) -> ()  [unwired: 8 out]
